vi "3D Cross Product.vi"(9 "B":T1, 10 "A":T1) -> (2 "A x B":T1)   [LabVIEW 2017]
uses:
  3D Point.ctl
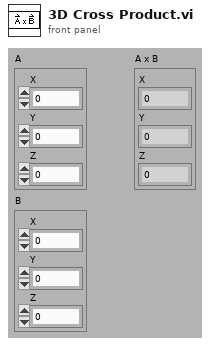
[diagram p1: front panel]
types:
  T1 = typedef "3D Point.ctl" = cluster{"X":dbl, "Y":dbl, "Z":dbl}
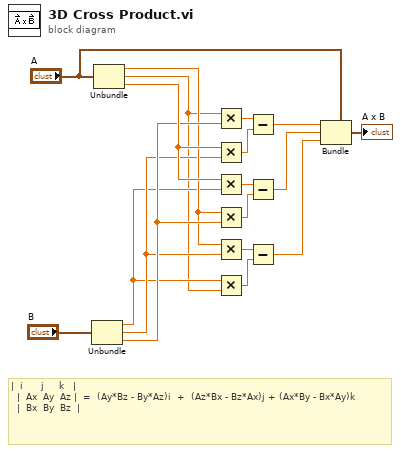
[diagram p0: block diagram]
diagram:
  # "|  i      j     k   |  \n  |  Ax  Ay  Az |  =  (Ay*Bz - By*Az)i  +  (Az*Bx - Bz*Ax)j + (Ax*By - Bx*Ay)k  \n  |  Bx  By  Bz  |"
  n1 = Unbundle("B") -> ("X"=w5:dbl, "Y"=w6:dbl, "Z"=w11:dbl)
  n2 = Unbundle("A") -> ("X"=w7:dbl, "Y"=w4:dbl, "Z"=w12:dbl)
  n3 = Multiply(x=w4, y=w11) -> (x*y=w15:dbl)
  n4 = Multiply(x=w12, y=w6) -> (x*y=w13:dbl)
  n5 = Multiply(x=w12, y=w5) -> (x*y=w10:dbl)
  n6 = Multiply(x=w7, y=w11) -> (x*y=w8:dbl)
  n7 = Multiply(x=w7, y=w6) -> (x*y=w3:dbl)
  n8 = Multiply(x=w5, y=w4) -> (x*y=w2:dbl)
  n9 = Subtract(x=w15, y=w13) -> (x-y=w14:dbl)
  n10 = Subtract(x=w10, y=w8) -> (x-y=w9:dbl)
  n11 = Subtract(x=w3, y=w2) -> (x-y=w1:dbl)
  n12 = Bundle(cluster="A", "X"=w14, "Y"=w9, "Z"=w1) -> (→"A x B":T1)
